vi "Cylinder Display.vi"(8 "error In":errorcluster, 11 "Sequence Context":refnum<k7>) -> (0 "error out":errorcluster)   [LabVIEW 2021, in "TestExec.lvclass"]
doc: "Use this template to build a simple state machine design pattern. Each state executes code and determines which state to transition to."
uses:
  TestExec.lvclass
  <vilib>/addons/TestStand/_TSUtility.llb/TestStand - Get Property Value (Number {Signed 32-bit Integer}).vi
  <vilib>/addons/TestStand/_TSUtility.llb/TestStand - Get Property Value (Boolean).vi
panel:
  in  "Image Array":string[](array[string])=["Retract All", "DMM Expand", "ACIR Expand", "HiPOT#1 Expand", "HIPOT#2 Expand"]
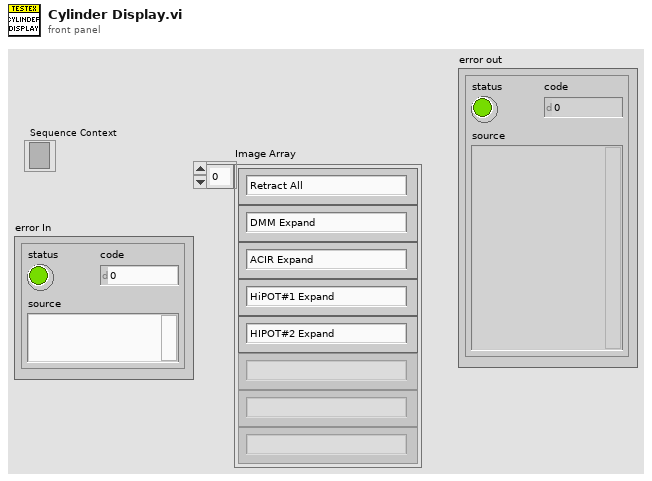
[diagram p1: front panel]
types:
  T1 = typedef "TestStand - Status Monitor.ctl" = cluster{"Sequence Context":refnum<k7>, "Execution":refnum<k7>, "Termination Monitor":refnum<k7>}
  T2 = typedef "imagedata.ctl" = cluster{"image type":i32, "image depth":i32, "image":u8[], "mask":u8[], "colors":u32[], "Rectangle":cluster{"left":i16, "top":i16, "right":i16, "bottom":i16}}
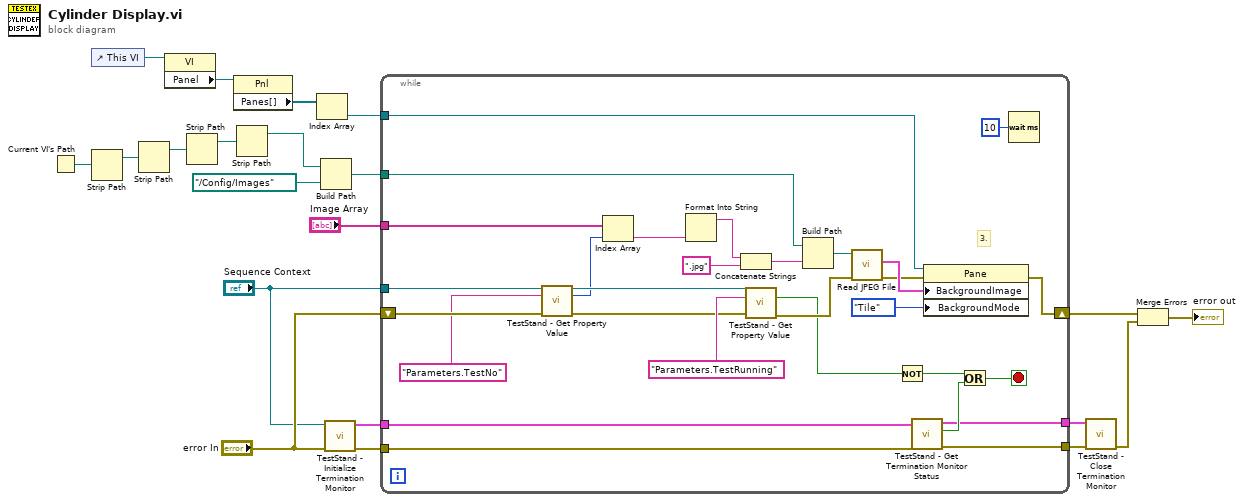
[diagram p0: block diagram]
diagram:
  n1 = Current VI's Path() -> (path=w17:path)
  n2 = control-ref of="This VI"() -> (w21:refnum<vi>)
  n3 = Strip Path(path=w17) -> (stripped path=w15:path)  [unwired: 1 out]
  n4 = Strip Path(path=w15) -> (stripped path=w14:path)  [unwired: 1 out]
  n5 = property class="VI"(reference=w21) -> ("Panel"=w20:refnum<vi>)  [unwired: 1 in, 2 out]
  n6 = Strip Path(path=w14) -> (stripped path=w13:path)  [unwired: 1 out]
  n7 = property class="Pnl"(reference=w20) -> ("Panes[]"=w19:refnum<vi>[])  [unwired: 1 in, 2 out]
  n8 = Strip Path(path=w13) -> (stripped path=w12:path)  [unwired: 1 out]
  n9 = Index Array(array=w19) -> (element=w18:refnum<vi>)  [unwired: 1 in]
  n10 = Build Path(base path=w12, name or relative path=path "../Config/Images") -> (appended path=w11:path)
  n11 = call <vilib>:"TestStand - Initialize Termination Monitor.vi"("error in (no error)"="error In", "Sequence Context In"="Sequence Context") -> ("error out"=w6:errorcluster, "Status Monitor Out"=w5:T1)  [unwired: 8 in]
  n12 = while {
    tunnel: w11 -> [w49]
    tunnel: w18 -> [w48]
    shift-right: [w50] -> w10
    shift-left: "error In" -> [w38]
    tunnel: "Image Array" -> [w40]
    tunnel: "Sequence Context" -> [w37]
    tunnel: w6 -> [w29]
    tunnel: w5 -> [w28]
    tunnel: [w25] -> w2
    tunnel: [w24] -> w3
    stop <- w27 stop-if-true
    # "3."
    n13 = call-poly <vilib>:"TestStand - Get Property Value.vi"("Sequence Context In"=w37, "Lookup String"="Parameters.TestNo", "error in (no error)"=w38) -> ("Sequence Context Out"=w35:refnum<k7>, "Value"=w22:i32, "error out"=w33:errorcluster)  [unwired: 10 in]
    n14 = Index Array(array=w40, index=w22) -> (element=w39:string)
    n15 = Format Into String(w39) -> (resulting string=w41:string)  [unwired: 3 in, 1 out]
    n16 = Concatenate Strings(w41, ".jpg" ("string")) -> (w44:string)
    n17 = call-poly <vilib>:"TestStand - Get Property Value.vi"("Sequence Context In"=w35, "Lookup String"="Parameters.TestRunning", "error in (no error)"=w33) -> ("Value"=w31:bool, "error out"=w32:errorcluster)  [unwired: 10 in, 1 out]
    n18 = Build Path(base path=w49, name or relative path=w44) -> (appended path=w47:path)
    n19 = call <vilib>:"Read JPEG File.vi"("error in (no error)"=w32, "path to JPEG file"=w47) -> ("error out"=w42:errorcluster, "image data"=w46:T2)  [unwired: 7 in, 1 out]
    n20 = Not(x=w31) -> (.not. x?=w30:bool)
    n21 = call <vilib>:"TestStand - Get Termination Monitor Status.vi"("error in (no error)"=w29, "Status Monitor In"=w28) -> ("error out"=w25:errorcluster, "Terminating or Aborting"=w26:bool, "Status Monitor Out"=w24:T1)  [unwired: 7 in]
    n22 = property class="Pane"(reference=w48, error in=w42, "BackgroundImage"=w46, "BackgroundMode"=enum16{"Stretch", "Center", "Tile"}."Tile" ("Background Mode")) -> (error out=w50:errorcluster)  [unwired: 1 out]
    n23 = Or(x=w30, y=w26) -> (x .or. y?=w27:bool)
    n24 = Wait (ms)(milliseconds to wait=u32 10) -> ()  [unwired: 1 out]
  }
  n25 = call <vilib>:"TestStand - Close Termination Monitor.vi"("error in (no error)"=w2, "Status Monitor In"=w3) -> ("error out"=w1:errorcluster)  [unwired: 9 in]
  n26 = Merge Errors(w10, w1) -> (→"error out":errorcluster)
